vi "Get Physical Image.vi"(7 "Delay(milliseconds)":i32=250, 8 "error in":errorcluster, 9 "Image In":T2, 10 "Camera Name":string, 11 "Gantry in":refnum<class "Gantry.lvclass">) -> (0 "error out":errorcluster, 2 "Physical Image":T1, 3 "Gantry out":refnum<class "Gantry.lvclass">)   [LabVIEW 2024, in "Gantry.lvclass"]
uses:
  Gantry.lvclass
  <vilib>/vision/Image Controls.llb/IMAQ Image.ctl
  Utils/Type Definitions/Physical Image.ctl
  Vec3d Class/Vec3d.lvclass
  Gantry.lvclass/Gantry.ctl
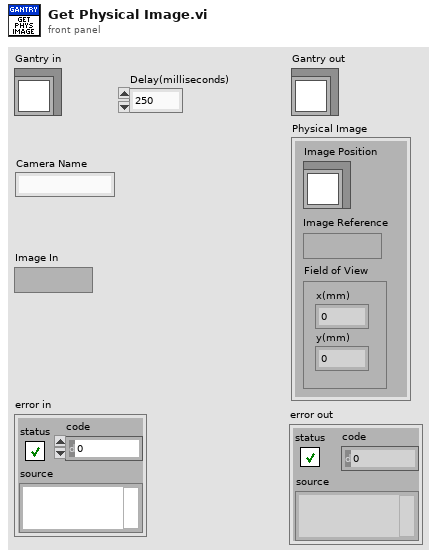
[diagram p1: front panel]
types:
  T1 = typedef "Physical Image.ctl" = cluster{"Image Position":refnum<class "Vec3d.lvclass">, "Image Reference":T2, "Field of View":cluster{"x(mm)":dbl, "y(mm)":dbl}}
  T2 = typedef "IMAQ Image.ctl" = refnum<image>
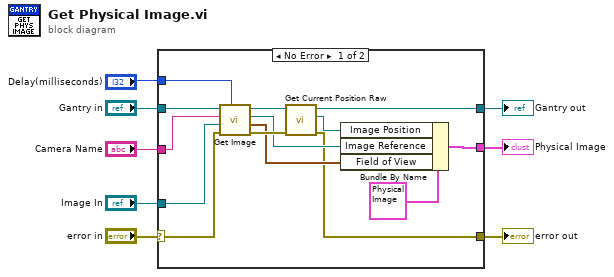
[diagram p0: block diagram]
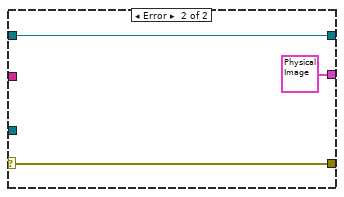
[diagram p2: hidden frame]
diagram:
  n1 = case shown="No Error" "error in" {
    selector: "error in" -> [w17 w25]
    tunnel: [w9 w25] -> w7
    tunnel: [w15 w24] -> w5
    tunnel: "Gantry in" -> [w22 w24]
    tunnel: "Image In" -> [w14 _]
    tunnel: [w12 T1 {"Image Position"=refnum, "Image Reference"=refnum, "Field of View"={"x(mm)"=0.0, "y(mm)"=0.0}} ("Physical Image")] -> w3
    tunnel: "Camera Name" -> [w10 _]
    tunnel: "Delay(milliseconds)" -> [w11 _]
    frame No Error {
      n2 = call-dynamic "Get Image.vi"("Delay(milliseconds)"=w11, "error in"=w17, "Image In"=w14, "Camera Name"=w10, "Gantry in"=w22) -> ("error out"=w21:errorcluster, "Field of View"=w13:cluster{"x-mm":dbl, "y-mm":dbl}, "Image Out"=w18:T2, "Gantry out"=w20:refnum<class "Gantry.lvclass">)  [unwired: 3 in]
      n3 = call-dynamic "Get Current Position Raw.vi"("error in"=w21, "Gantry in"=w20) -> ("error out"=w9:errorcluster, "Vec3d Class out"=w16:refnum<class "Vec3d.lvclass">, "Gantry out"=w15:refnum<class "Gantry.lvclass">)  [unwired: 7 in]
      n4 = Bundle By Name(cluster=T1 {"Image Position"=refnum, "Image Reference"=refnum, "Field of View"={"x(mm)"=0.0, "y(mm)"=0.0}} ("Physical Image"), "Image Position"=w16, "Image Reference"=w18, "Field of View"=w13) -> (w12:T1)
    }
    frame Error {
    }
  }
  "error out" <- w7
  "Gantry out" <- w5
  "Physical Image" <- w3
